vi "testcase - INI-Static-Variable-Support.vi"() -> ()   [LabVIEW 2017]
uses:
  <userlib>/_NEVSTOP/Communicable State Machine(CSM)/Communicable State Machine.lvlib
  INI-Static-Variable-Support/INI-Static-Variable-Support.lvlib
panel:
  out "error out 2":errorcluster
  out "States with configuration from ini file 2":string="Data: Load Configuration >> ip:https:%2F%2Fwww.ni.com;port:443 -> NetworkModule\r\nData: Load Configuration >> https:%2F%2Fwww.ni.com:443 -> NetworkModule\r\nData: Load Configuration >> ip:https:%2F%2Fwww.ni.com -> NetworkModule\r\nData: Load Configuration >> 443 -> NetworkModule"
  in  "States with ${Variable} 2":string="Data: Load Configuration >> ip:${ip:127.0.0.1};port:${port:5000} -> NetworkModule\nData: Load Configuration >> ${ip:127.0.0.1}:${port:5000} -> NetworkModule\nData: Load Configuration >> ip:${ip} -> NetworkModule\nData: Load Configuration >> ${port:5000} -> NetworkModule"
  in  "States with ${Variable}":string="Data: Load Configuration >> ip:${ip:127.0.0.1};port:${port:5000} -> NetworkModule\nData: Load Configuration >> ${ip:127.0.0.1}:${port:5000} -> NetworkModule\nData: Load Configuration >> ip:${ip} -> NetworkModule\nData: Load Configuration >> ${port:5000} -> NetworkModule"
  out "States with configuration from ini file":string="Data: Load Configuration >> ip:https:%2F%2Fwww.ni.com;port:443 -> NetworkModule\r\nData: Load Configuration >> https:%2F%2Fwww.ni.com:443 -> NetworkModule\r\nData: Load Configuration >> ip:https:%2F%2Fwww.ni.com -> NetworkModule\r\nData: Load Configuration >> 443 -> NetworkModule"
  out "error out":errorcluster
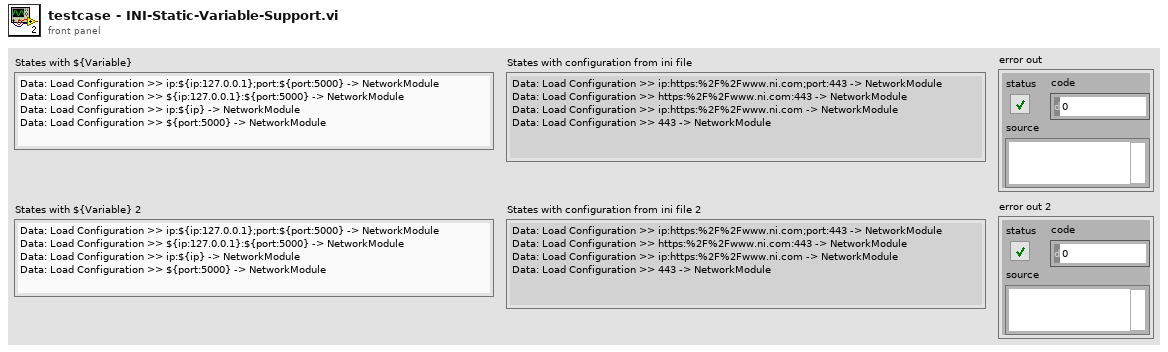
[diagram p1: front panel]
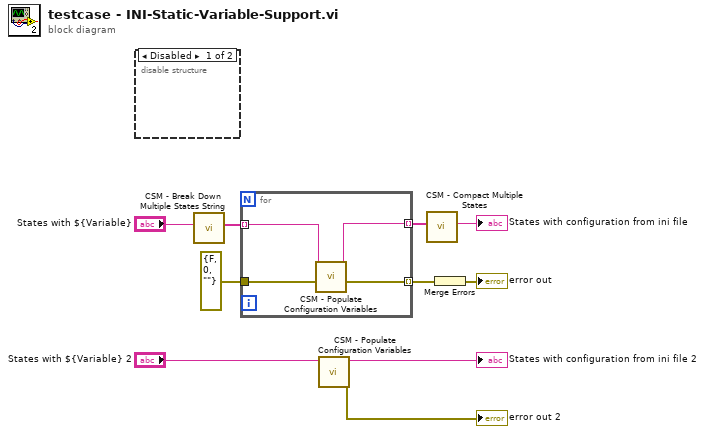
[diagram p0: block diagram]
diagram:
  n1 = disable-structure shown="Disabled" {
    frame Disabled {
    }
    frame Enabled {
    }
  }
  n2 = call <userlib>:"CSM - Break Down Multiple States String.vi"("States"="States with ${Variable}") -> ("Multiple States"=w5:string[])  [unwired: 10 in]
  n3 = for {
    tunnel: [w14] -> w9 mode=indexing
    tunnel: w5 -> [w13] mode=indexing
    tunnel: errorcluster {"status"=FALSE, "code"=0, "source"=""} ("error out") -> [w12]
    tunnel: [w11] -> w10 mode=indexing
    n4 = call "CSM - Populate Configuration Variables.vi"("error in (no error)"=w12, "String in"=w13) -> ("error out"=w11:errorcluster, "String out"=w14:string)  [unwired: 6 in]
  }
  n5 = call "CSM - Populate Configuration Variables.vi"("String in"="States with ${Variable} 2") -> ("error out"=→"error out 2":errorcluster, "String out"=→"States with configuration from ini file 2":string)  [unwired: 7 in]
  n6 = call <userlib>:"CSM - Compact Multiple States.vi"("Multiple States"=w9) -> ("States"=→"States with configuration from ini file":string)  [unwired: 9 in]
  n7 = Merge Errors(w10) -> (→"error out":errorcluster)
